vi "Restore Startup Configuration.vi"(8 "error in (no error)":errorcluster, 10 "Startup Configuration File":path=path "C:/Data/Config/start-up.cfg", 11 "Monitor-Pulse in":refnum<class "Monitor-Pulse.lvclass">) -> (0 "error out":errorcluster, 3 "Monitor-Pulse out":refnum<class "Monitor-Pulse.lvclass">)   [LabVIEW 2015, in "Monitor-Pulse.lvclass"]
uses:
  Monitor-Pulse.lvclass
  Start-up Configuration.ctl
  Module Types.ctl
  Monitor-Pulse.lvclass/Monitor-Pulse.ctl
  <vilib>/Utility/error.llb/Error Cluster From Error Code.vi
  <vilib>/ErrorRing/Error Ring.xnode
  <vilib>/Utility/config.llb/NI_LVConfig.lvlib
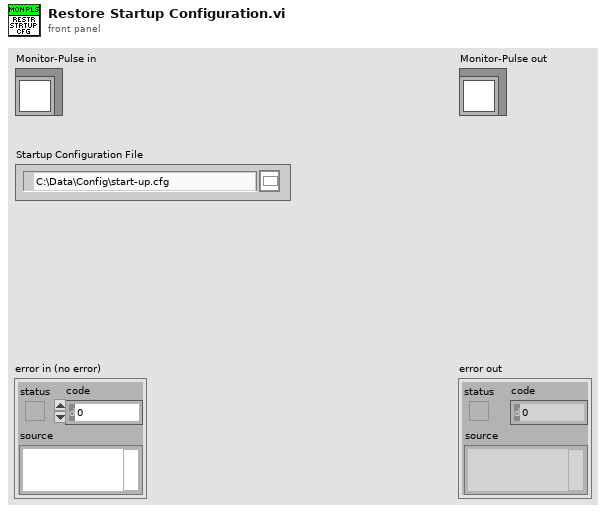
[diagram p1: front panel]
types:
  T1 = typedef "NI_LVConfig.lvlib/Config Data RefNum.ctl" = refnum<k1>
  T2 = typedef "Start-up Configuration.ctl" = cluster{"Load Modules":T3[]}
  T3 = typedef "Module Types.ctl" = enum16{"NONE", "NI-DAQmx", "NI-Scope", "Red Pitaya Digitizer", "GaGe", "VISA Device", "Red Piataya Lockin", "Monitor Controller", "Pulse Controller", "Integrate Pulse"}
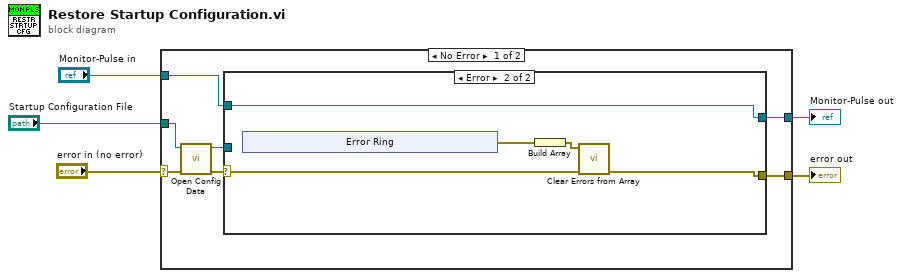
[diagram p0: block diagram]
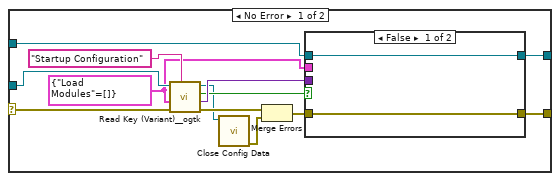
[diagram p2: hidden frame]
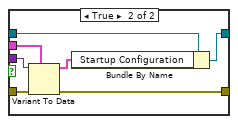
[diagram p3: hidden frame]
diagram:
  n1 = case shown="No Error" "error in (no error)" {
    selector: "error in (no error)" -> [w8 w45]
    tunnel: [w7 w45] -> w4
    tunnel: [w9 w44] -> w2
    tunnel: "Monitor-Pulse in" -> [w12 w44]
    tunnel: "Startup Configuration File" -> [w11 _]
    frame No Error {
      n2 = call <vilib>:"Open Config Data.vi"("error in (no error)"=w8, "configuration file path"=w11) -> ("error out"=w6:errorcluster, "refnum"=w10:T1)  [unwired: 7 in, 1 out]
      n3 = case shown="Error" w6 {
        selector: w6 -> [w13 w39]
        tunnel: w12 -> [w25 w38]
        tunnel: w10 -> [w23 _]
        tunnel: [w22 w38] -> w9
        tunnel: [w19 w37] -> w7
        frame No Error {
          w20 = T2 {"Load Modules"=[]} ("Initial Configuration")
          n4 = call <userlib>:"Read Key (Variant)__ogtk.vi"("section"="Startup Configuration", "error in (no error)"=w13, "type"=w20, "refnum"=w23) -> ("error out"=w17:errorcluster, "key-value"=w21:variant, "found?"=w18:bool, "refnum out"=w16:T1)  [unwired: 4 in]
          n5 = call <vilib>:"Close Config Data.vi"("refnum"=w16) -> ("error out"=w15:errorcluster)  [unwired: 9 in, 1 out]
          n6 = Merge Errors(w17, w15) -> (w14:errorcluster)
          n7 = case shown="False" w18 {
            tunnel: w25 -> [w27 w34]
            tunnel: [w27 w33] -> w22
            tunnel: w14 -> [w26 w32]
            tunnel: w21 -> [_ w31]
            tunnel: w20 -> [_ w30]
            tunnel: [w26 w28] -> w19
            frame False {
            }
            frame True {
              n8 = Variant To Data(error in=w32, type=w30, Variant=w31) -> (data=w29:T2, error out=w28:errorcluster)
              n9 = Bundle By Name(cluster=w34, "Startup Configuration"=w29) -> (w33:refnum<class "Monitor-Pulse.lvclass">)
            }
          }
        }
        frame Error {
          n10 = xnode "Error Ring"() -> ("error out"=w36:errorcluster)
          n11 = Build Array(w36) -> (w35:errorcluster[])
          n12 = call "Clear Errors from Array.vi"("Error In"=w39, "Errors to clear"=w35) -> ("Error Out"=w37:errorcluster)  [unwired: 8 in, 1 out]
        }
      }
    }
    frame Error {
    }
  }
  "error out" <- w4
  "Monitor-Pulse out" <- w2
